vi "OP1_RISCALDO.vi"(0 "Esito 2 in":cluster{"Si":bool, "No":bool}, 1 "Esito 3 in":cluster{"Si":bool, "No":bool}, 2 "Esito 4 in":cluster{"Si":bool, "No":bool}, 3 "Esito 5 in":cluster{"Si":bool, "No":bool}, 4 "Esito 6 in":cluster{"Si":bool, "No":bool}, 5 "Esito 7 in":cluster{"Si":bool, "No":bool}, 6 "Esito 8 in":cluster{"Si":bool, "No":bool}, 7 "Esito 9 in":cluster{"Si":bool, "No":bool}, 8 "Esito 1 in":cluster{"Si":bool, "No":bool}, 9 "Tasto premuto":T1(array[ring]), 10 "Tipo specifica":string, 12 "Stato in":u16, 14 "Stato out":u16) -> (16 "Dato":string[](array[string]), 17 "ANNULLA PROVA":bool, 18 "Esito 1 out":T2, 19 "i out":i32=1, 20 "Esito 2 out":T2, 21 "Esito 3 out":T2, 22 "Esito 4 out":T2, 23 "Esito 5 out":T2, 24 "Esito 6 out":T2, 25 "Esito 7 out":T2, 26 "Esito 8 out":T2, 27 "Esito 9 out":T2)   [LabVIEW 2022 SP3]
uses:
  Labview/Globali.vi
panel:
  out "Memoria fase succ":bool
  in  "i max":i32
  in  "i":i32=1
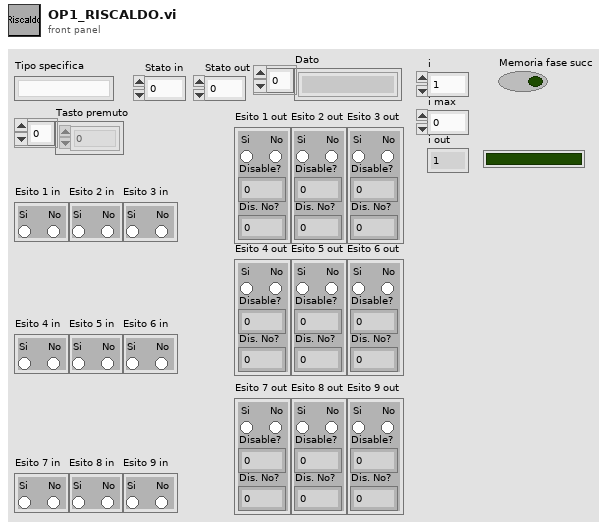
[diagram p1: front panel]
types:
  T1 = enum16{"0", "1", "2", "3", "4", "5", "6", "7", "8", "9", "A", "B", "C", "D", "E", "F", "G", "H", "I", "J", "K", "L", "M", "N", "O", "P", "Q", "R", "S", "T", "U", "V", "W", "X", "Y", "Z", "F1", "F2", "F3", "F4", "F5", "F6", "F7", "F8", "F9", "F10", "F11", "F12", "F13", "F14", "F15", "ADD", "BACK", "BACKSLASH", "CAPITAL", "COMMA", "DECIMAL", "DELETE", "DIVIDE", "DOWN", "END", "EQUALS", "ESCAPE", "GRAVE (`)", "HOME", "INSERT", "LBRACKET", "LCONTROL", "LEFT", "L ALT", "LSHIFT", "LWIN", "MINUS", "MULTIPLY", "NEXT", "NUMLOCK", "NUMPAD_0", "NUMPAD_1", "NUMPAD_2", "NUMPAD_3", "NUMPAD_4", "NUMPAD_5", "NUMPAD_6", "NUMPAD_7", "NUMPAD_8", "NUMPAD_9", "PAUSE", "PERIOD", "PRIOR (PG UP)", "RBRACKET", "RCONTROL", "RETURN", "RIGHT", "R ALT", "RSHIFT", "RWIN", "SCROLL", "SEMICOLON", "SLASH", "SPACE", "SUBTRACT", "TAB", "UP", "ENTER (num pad)", "' (quote)"}[]
  T2 = cluster{"Disable?":i16, "Si":bool, "No":bool, "Dis. No?":i16}
  T3 = cluster{"Esito 1 out":cluster{"Disable?":i16, "Si":bool, "No":bool, "Dis. No?":i16}, "Esito 2 out":cluster{"Disable?":i16, "Si":bool, "No":bool, "Dis. No?":i16}, "Esito 3 out":cluster{"Disable?":i16, "Si":bool, "No":bool, "Dis. No?":i16}, "Esito 4 out":cluster{"Disable?":i16, "Si":bool, "No":bool, "Dis. No?":i16}, "Esito 5 out":cluster{"Disable?":i16, "Si":bool, "No":bool, "Dis. No?":i16}, "Esito 6 out":cluster{"Disable?":i16, "Si":bool, "No":bool, "Dis. No?":i16}, "Esito 7 out":cluster{"Disable?":i16, "Si":bool, "No":bool, "Dis. No?":i16}, "Esito 8 out":cluster{"Disable?":i16, "Si":bool, "No":bool, "Dis. No?":i16}, "Esito 9 out":cluster{"Disable?":i16, "Si":bool, "No":bool, "Dis. No?":i16}}
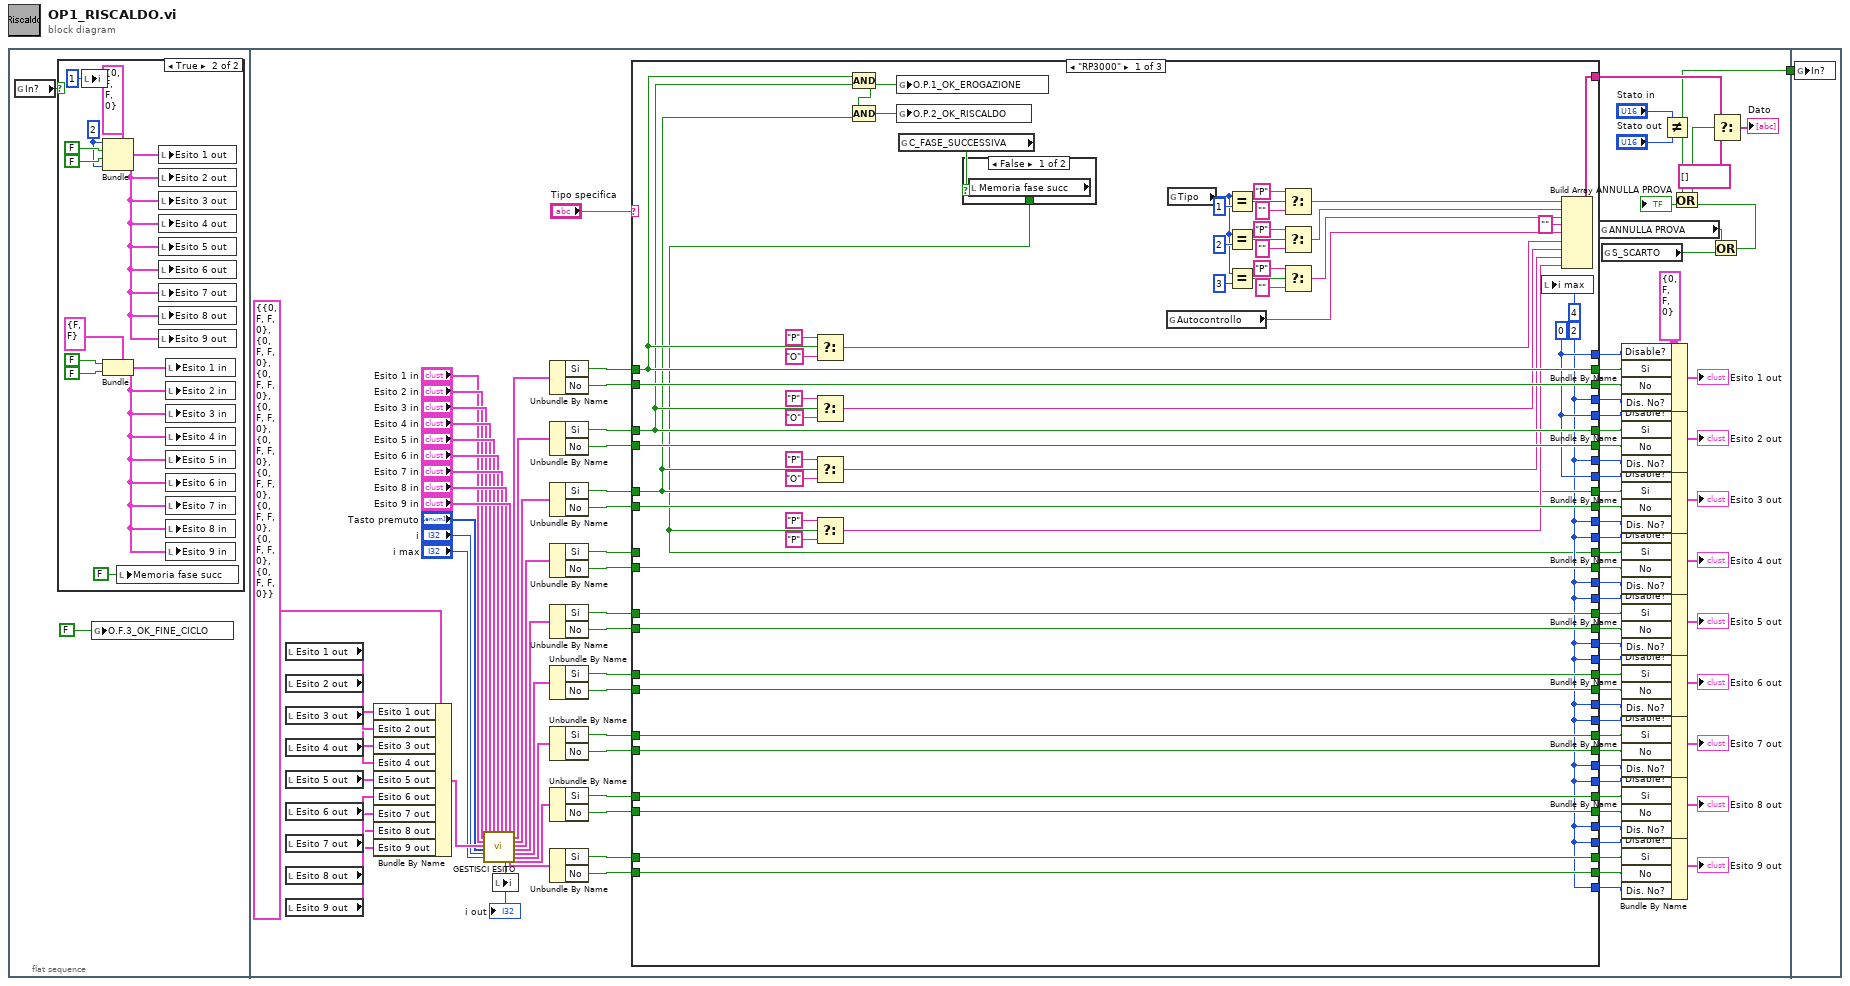
[diagram p0: block diagram]
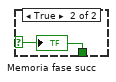
[diagram p3: hidden frame]
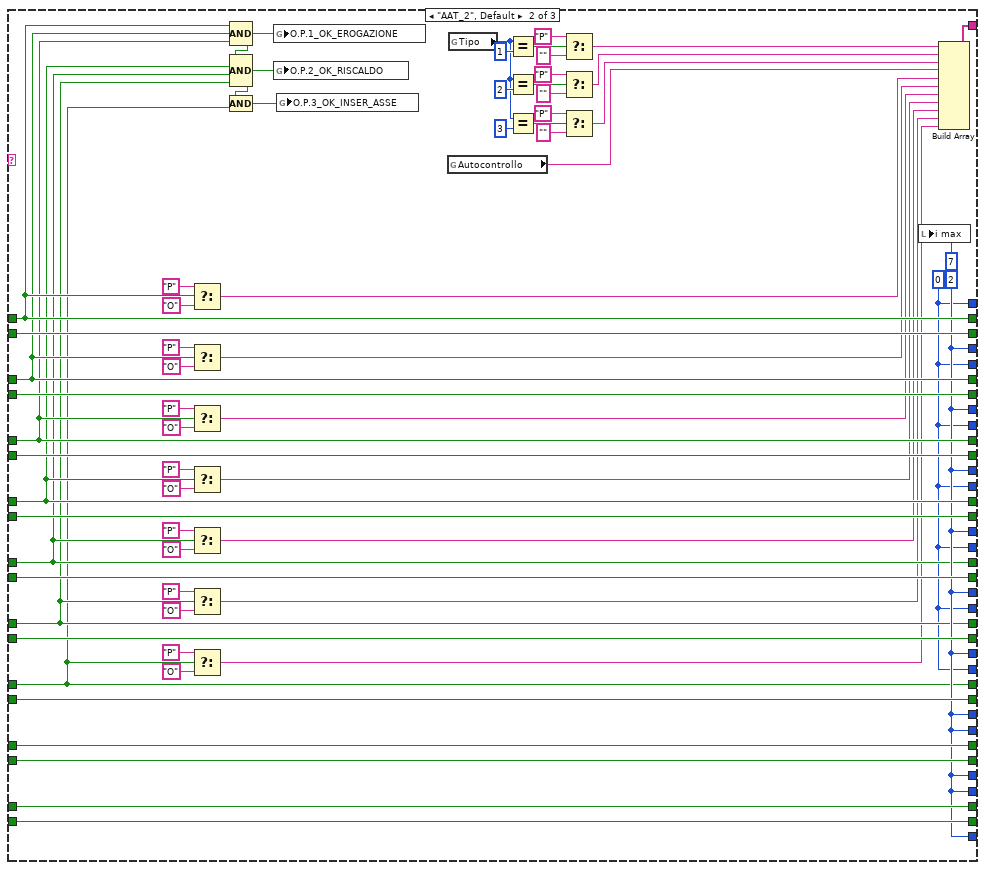
[diagram p4: hidden frame]
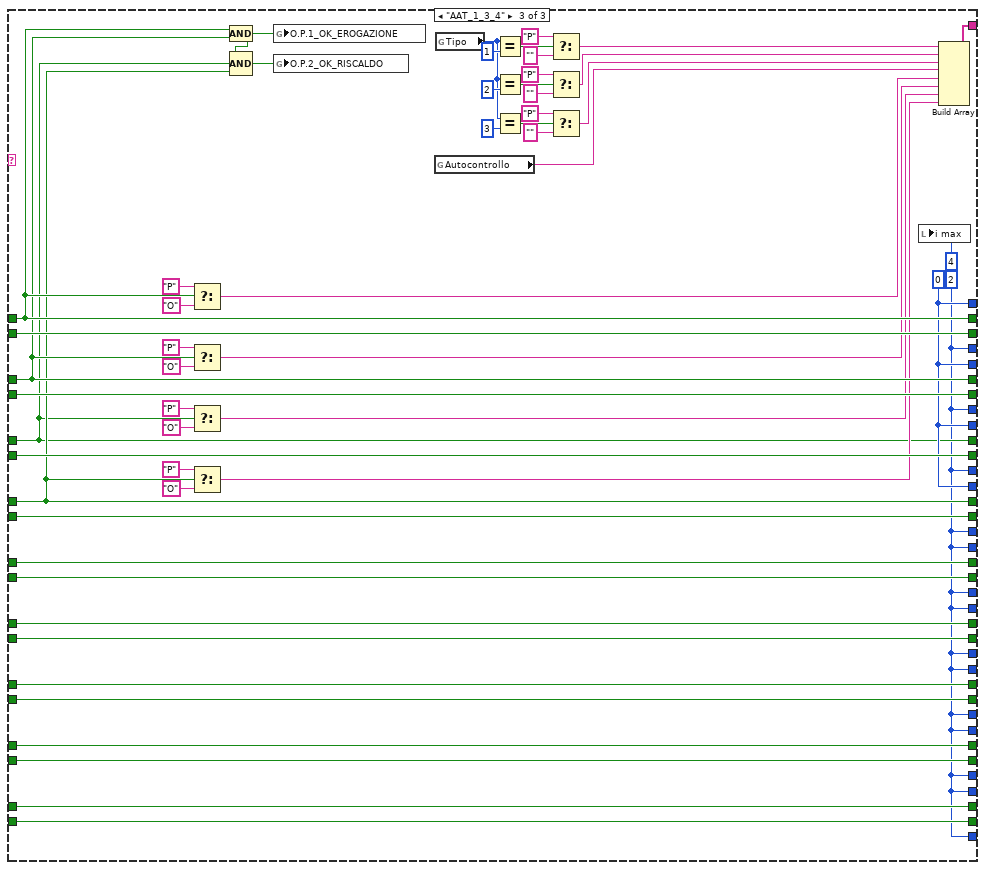
[diagram p5: hidden frame]
diagram:
  n1 = flat-sequence {
    tunnel: [w19] -> w1
    tunnel: w1 -> [w296]
    frame #0 {
      n2 = global read "Globali.vi" "In?"() -> (w3:bool)
      n3 = case shown="True" w3 {
        frame False {
        }
        frame True {
          w11 = i16 2 ("Disable?")
          n4 = local write "i"(1 ("i")) -> ()
          n5 = Bundle(cluster=T2 {"Disable?"=0, "Si"=FALSE, "No"=FALSE, "Dis. No?"=0} ("Esito 1 out"), "Disable?"=w11, "Si"=FALSE, "No"=FALSE, "Dis. No?"=w11) -> (w10:T2)
          n6 = Bundle(cluster=cluster{"Si":bool, "No":bool} {"Si"=FALSE, "No"=FALSE} ("Esito 1 in"), "Si"=FALSE, "No"=FALSE) -> (w8:cluster{"Si":bool, "No":bool})
          n7 = local write "Memoria fase succ"(FALSE ("Memoria fase succ")) -> ()
          n8 = local write "Esito 1 out"(w10) -> ()
          n9 = local write "Esito 2 out"(w10) -> ()
          n10 = local write "Esito 3 out"(w10) -> ()
          n11 = local write "Esito 4 out"(w10) -> ()
          n12 = local write "Esito 5 out"(w10) -> ()
          n13 = local write "Esito 6 out"(w10) -> ()
          n14 = local write "Esito 7 out"(w10) -> ()
          n15 = local write "Esito 8 out"(w10) -> ()
          n16 = local write "Esito 9 out"(w10) -> ()
          n17 = local write "Esito 1 in"(w8) -> ()
          n18 = local write "Esito 2 in"(w8) -> ()
          n19 = local write "Esito 3 in"(w8) -> ()
          n20 = local write "Esito 4 in"(w8) -> ()
          n21 = local write "Esito 5 in"(w8) -> ()
          n22 = local write "Esito 6 in"(w8) -> ()
          n23 = local write "Esito 7 in"(w8) -> ()
          n24 = local write "Esito 8 in"(w8) -> ()
          n25 = local write "Esito 9 in"(w8) -> ()
        }
      }
      n26 = global write "Globali.vi" "O.F.3_OK_FINE_CICLO"(FALSE ("O.F.3_OK_FINE_CICLO")) -> ()
    }
    frame #1 {
      w62 = T2 {"Disable?"=0, "Si"=FALSE, "No"=FALSE, "Dis. No?"=0} ("Esito 1 out")
      n27 = local read "Esito 1 out"() -> (w51:T2)
      n28 = local read "Esito 2 out"() -> (w50:T2)
      n29 = local read "Esito 3 out"() -> (w49:T2)
      n30 = local read "Esito 4 out"() -> (w48:T2)
      n31 = local read "Esito 5 out"() -> (w47:T2)
      n32 = local read "Esito 6 out"() -> (w46:T2)
      n33 = local read "Esito 7 out"() -> (w45:T2)
      n34 = local read "Esito 8 out"() -> (w44:T2)
      n35 = local read "Esito 9 out"() -> (w43:T2)
      n36 = Bundle By Name(cluster=T3 {"Esito 1 out"={"Disable?"=0, "Si"=FALSE, "No"=FALSE, "Dis. No?"=0}, "Esito 2 out"={"Disable?"=0, "Si"=FALSE, "No"=FALSE, "Dis. No?"=0}, "Esito 3 out"={"Disable?"=0, "Si"=FALSE, "No"=FALSE, "Dis. No?"=0}, "Esito 4 out"={"Disable?"=0, "Si"=FALSE, "No"=FALSE, "Dis. No?"=0}, "Esito 5 out"={"Disable?"=0, "Si"=FALSE, "No"=FALSE, "Dis. No?"=0}, "Esito 6 out"={"Disable?"=0, "Si"=FALSE, "No"=FALSE, "Dis. No?"=0}, "Esito 7 out"={"Disable?"=0, "Si"=FALSE, "No"=FALSE, "Dis. No?"=0}, "Esito 8 out"={"Disable?"=0, "Si"=FALSE, "No"=FALSE, "Dis. No?"=0}, "Esito 9 out"={"Disable?"=0, "Si"=FALSE, "No"=FALSE, "Dis. No?"=0}} ("Cluster"), "Esito 1 out"=w51, "Esito 2 out"=w50, "Esito 3 out"=w49, "Esito 4 out"=w48, "Esito 5 out"=w47, "Esito 6 out"=w46, "Esito 7 out"=w45, "Esito 8 out"=w44, "Esito 9 out"=w43) -> (w42:T3)
      n37 = call "GESTISCI ESITO.vi"("Esito 3 in"="Esito 3 in", "Esito 2 in"="Esito 2 in", "Esito 1 in"="Esito 1 in", "Cluster"=w42, "Tasto premuto"="Tasto premuto", "i in"="i", "i max"="i max", "Esito 4 in"="Esito 4 in", "Esito 5 in"="Esito 5 in", "Esito 6 in"="Esito 6 in", "Esito 7 in"="Esito 7 in", "Esito 8 in"="Esito 8 in", "Esito 9 in"="Esito 9 in") -> ("i out"=w20:i32, "Esito 9 in 2"=w21:cluster{"Si":bool, "No":bool}, "Esito 1 in 2"=w29:cluster{"Si":bool, "No":bool}, "Esito 2 in 2"=w28:cluster{"Si":bool, "No":bool}, "Esito 3 in 2"=w27:cluster{"Si":bool, "No":bool}, "Esito 4 in 2"=w26:cluster{"Si":bool, "No":bool}, "Esito 5 in 2"=w25:cluster{"Si":bool, "No":bool}, "Esito 6 in 2"=w24:cluster{"Si":bool, "No":bool}, "Esito 7 in 2"=w23:cluster{"Si":bool, "No":bool}, "Esito 8 in 2"=w22:cluster{"Si":bool, "No":bool})  [unwired: 5 in]
      "i out" <- w20
      n38 = local write "i"(w20) -> ()
      n39 = Unbundle By Name(w29) -> ("Si"=w86:bool, "No"=w85:bool)
      n40 = Unbundle By Name(w28) -> ("Si"=w69:bool, "No"=w70:bool)
      n41 = Unbundle By Name(w27) -> ("Si"=w71:bool, "No"=w72:bool)
      n42 = Unbundle By Name(w26) -> ("Si"=w73:bool, "No"=w74:bool)
      n43 = Unbundle By Name(w25) -> ("Si"=w75:bool, "No"=w76:bool)
      n44 = Unbundle By Name(w24) -> ("Si"=w77:bool, "No"=w78:bool)
      n45 = Unbundle By Name(w23) -> ("Si"=w79:bool, "No"=w80:bool)
      n46 = Unbundle By Name(w22) -> ("Si"=w81:bool, "No"=w82:bool)
      n47 = Unbundle By Name(w21) -> ("Si"=w83:bool, "No"=w84:bool)
      n48 = case shown="\"RP3000\"" "Tipo specifica" {
        tunnel: [w152 w214 w272] -> w66
        tunnel: [w146 w198 w264] -> w113
        tunnel: [w146 w198 w264] -> w112
        tunnel: [w146 w198 w264] -> w111
        tunnel: [w143 w198 w264] -> w110
        tunnel: [w143 w198 w261] -> w109
        tunnel: [w143 w198 w261] -> w108
        tunnel: [w143 w198 w261] -> w107
        tunnel: [w143 w215 w261] -> w106
        tunnel: [w143 w215 w261] -> w105
        tunnel: [w161 w228 w281] -> w104
        tunnel: [w160 w227 w280] -> w103
        tunnel: [w159 w226 w279] -> w102
        tunnel: [w162 w229 w282] -> w101
        tunnel: [w145 w219 w262] -> w100
        tunnel: [w177 w242 w295] -> w99
        tunnel: [w141 w217 w263] -> w98
        tunnel: [w176 w241 w294] -> w97
        tunnel: [w144 w208 w267] -> w96
        tunnel: [w175 w240 w293] -> w95
        tunnel: [w174 w202 w266] -> w94
        tunnel: [w173 w239 w292] -> w93
        tunnel: [w172 w201 w265] -> w92
        tunnel: [w171 w238 w291] -> w91
        tunnel: [w170 w237 w290] -> w90
        tunnel: [w169 w236 w289] -> w89
        tunnel: [w168 w235 w288] -> w88
        tunnel: [w167 w234 w287] -> w87
        tunnel: w86 -> [w161 w228 w281]
        tunnel: w85 -> [w160 w227 w280]
        tunnel: w84 -> [w167 w234 w287]
        tunnel: w83 -> [w168 w235 w288]
        tunnel: w82 -> [w169 w236 w289]
        tunnel: w81 -> [w170 w237 w290]
        tunnel: w80 -> [w171 w238 w291]
        tunnel: w79 -> [w172 w201 w265]
        tunnel: w78 -> [w173 w239 w292]
        tunnel: w77 -> [w174 w202 w266]
        tunnel: w76 -> [w175 w240 w293]
        tunnel: w75 -> [w144 w208 w267]
        tunnel: w74 -> [w176 w241 w294]
        tunnel: w73 -> [_ w217 w263]
        tunnel: w72 -> [w177 w242 w295]
        tunnel: w71 -> [w145 w219 w262]
        tunnel: w70 -> [w162 w229 w282]
        tunnel: w69 -> [w159 w226 w279]
        tunnel: [w143 w215 w261] -> w61
        tunnel: [w143 w215 w261] -> w60
        tunnel: [w143 w215 w261] -> w59
        tunnel: [w143 w215 w261] -> w58
        tunnel: [w143 w215 w261] -> w57
        tunnel: [w143 w215 w261] -> w56
        tunnel: [w143 w215 w261] -> w55
        tunnel: [w143 w215 w261] -> w54
        tunnel: [w143 w215 w261] -> w53
        frame "RP3000" {
          w143 = 2
          w146 = 0
          n49 = Select(t="P", s=w161, f="O") -> (s? t:f=w148:string)
          n50 = Select(t="P", s=w159, f="O") -> (s? t:f=w149:string)
          n51 = Select(t="P", s=w145, f="O") -> (s? t:f=w150:string)
          n52 = Compound Arithmetic op=AND(w161, w159) -> (w154:bool)
          n53 = Compound Arithmetic op=AND(w154, w145) -> (w153:bool)
          n54 = global write "Globali.vi" "O.P.1_OK_EROGAZIONE"(w154) -> ()
          n55 = global write "Globali.vi" "O.P.2_OK_RISCALDO"(w153) -> ()
          n56 = global read "Globali.vi" "C_FASE_SUCCESSIVA"() -> (w142:bool)
          n57 = case shown="False" w142 {
            selector: w142 -> [_ w179]
            tunnel: [w178 w179] -> w141
            frame False {
              n58 = local read "Memoria fase succ"() -> (w178:bool)
            }
            frame True {
              "Memoria fase succ" <- w179
            }
          }
          n59 = Select(t="P", s=w141, f="P") -> (s? t:f=w151:string)
          n60 = global read "Globali.vi" "Autocontrollo"() -> (w127:string)
          n61 = global read "Globali.vi" "Tipo"() -> (w128:i16)
          n62 = Equal?(x=w128, y=i16 1) -> (x = y?=w137:bool)
          n63 = Equal?(x=w128, y=i16 2) -> (x = y?=w133:bool)
          n64 = Equal?(x=w128, y=i16 3) -> (x = y?=w132:bool)
          n65 = Select(t="P", s=w137, f="") -> (s? t:f=w124:string)
          n66 = Select(t="P", s=w133, f="") -> (s? t:f=w125:string)
          n67 = Select(t="P", s=w132, f="") -> (s? t:f=w126:string)
          n68 = local write "i max"(4) -> ()
          n69 = Build Array(w124, w125, w126, "" ("element"), w127, w148, w149, w150, w151) -> (w152:string[])
        }
        frame "AAT_2", Default {
          w215 = 2
          w198 = 0
          n70 = Select(t="P", s=w228, f="O") -> (s? t:f=w209:string)
          n71 = Select(t="P", s=w226, f="O") -> (s? t:f=w210:string)
          n72 = Select(t="P", s=w219, f="O") -> (s? t:f=w211:string)
          n73 = Select(t="P", s=w217, f="O") -> (s? t:f=w212:string)
          n74 = Select(t="P", s=w208, f="O") -> (s? t:f=w213:string)
          n75 = Select(t="P", s=w202, f="O") -> (s? t:f=w200:string)
          n76 = Select(t="P", s=w201, f="O") -> (s? t:f=w199:string)
          n77 = Compound Arithmetic op=AND(w228, w226, w219) -> (w218:bool)
          n78 = Compound Arithmetic op=AND(w218, w217, w208, w202) -> (w216:bool)
          n79 = Compound Arithmetic op=AND(w216, w201) -> (w207:bool)
          n80 = global write "Globali.vi" "O.P.1_OK_EROGAZIONE"(w218) -> ()
          n81 = global write "Globali.vi" "O.P.2_OK_RISCALDO"(w216) -> ()
          n82 = global write "Globali.vi" "O.P.3_OK_INSER_ASSE"(w207) -> ()
          n83 = global read "Globali.vi" "Autocontrollo"() -> (w180:string)
          n84 = global read "Globali.vi" "Tipo"() -> (w184:i16)
          n85 = Equal?(x=w184, y=i16 1) -> (x = y?=w193:bool)
          n86 = Equal?(x=w184, y=i16 2) -> (x = y?=w189:bool)
          n87 = Equal?(x=w184, y=i16 3) -> (x = y?=w188:bool)
          n88 = Select(t="P", s=w193, f="") -> (s? t:f=w183:string)
          n89 = Select(t="P", s=w189, f="") -> (s? t:f=w182:string)
          n90 = Select(t="P", s=w188, f="") -> (s? t:f=w181:string)
          n91 = local write "i max"(7) -> ()
          n92 = Build Array(w183, w182, w181, w180, w209, w210, w211, w212, w213, w200, w199) -> (w214:string[])
        }
        frame "AAT_1_3_4" {
          w261 = 2
          w264 = 0
          n93 = Select(t="P", s=w281, f="O") -> (s? t:f=w268:string)
          n94 = Select(t="P", s=w279, f="O") -> (s? t:f=w269:string)
          n95 = Select(t="P", s=w262, f="O") -> (s? t:f=w270:string)
          n96 = Select(t="P", s=w263, f="O") -> (s? t:f=w271:string)
          n97 = Compound Arithmetic op=AND(w281, w279) -> (w274:bool)
          n98 = Compound Arithmetic op=AND(w274, w262, w263) -> (w273:bool)
          n99 = global write "Globali.vi" "O.P.1_OK_EROGAZIONE"(w274) -> ()
          n100 = global write "Globali.vi" "O.P.2_OK_RISCALDO"(w273) -> ()
          n101 = global read "Globali.vi" "Autocontrollo"() -> (w243:string)
          n102 = global read "Globali.vi" "Tipo"() -> (w247:i16)
          n103 = Equal?(x=w247, y=i16 1) -> (x = y?=w256:bool)
          n104 = Equal?(x=w247, y=i16 2) -> (x = y?=w252:bool)
          n105 = Equal?(x=w247, y=i16 3) -> (x = y?=w251:bool)
          n106 = Select(t="P", s=w256, f="") -> (s? t:f=w246:string)
          n107 = Select(t="P", s=w252, f="") -> (s? t:f=w245:string)
          n108 = Select(t="P", s=w251, f="") -> (s? t:f=w244:string)
          n109 = local write "i max"(4) -> ()
          n110 = Build Array(w246, w245, w244, w243, w268, w269, w270, w271) -> (w272:string[])
        }
      }
      n111 = global read "Globali.vi" "ANNULLA PROVA"() -> (w16:bool)
      n112 = global read "Globali.vi" "S_SCARTO"() -> (w17:bool)
      n113 = Bundle By Name(cluster=w62, "Disable?"=w113, "Si"=w104, "No"=w103, "Dis. No?"=w61) -> (→"Esito 1 out":T2)
      n114 = Bundle By Name(cluster=w62, "Disable?"=w112, "Si"=w102, "No"=w101, "Dis. No?"=w60) -> (→"Esito 2 out":T2)
      n115 = Bundle By Name(cluster=w62, "Disable?"=w111, "Si"=w100, "No"=w99, "Dis. No?"=w59) -> (→"Esito 3 out":T2)
      n116 = Bundle By Name(cluster=w62, "Disable?"=w110, "Si"=w98, "No"=w97, "Dis. No?"=w58) -> (→"Esito 4 out":T2)
      n117 = Bundle By Name(cluster=w62, "Disable?"=w109, "Si"=w96, "No"=w95, "Dis. No?"=w57) -> (→"Esito 5 out":T2)
      n118 = Bundle By Name(cluster=w62, "Disable?"=w108, "Si"=w94, "No"=w93, "Dis. No?"=w56) -> (→"Esito 6 out":T2)
      n119 = Bundle By Name(cluster=w62, "Disable?"=w107, "Si"=w92, "No"=w91, "Dis. No?"=w55) -> (→"Esito 7 out":T2)
      n120 = Bundle By Name(cluster=w62, "Disable?"=w106, "Si"=w90, "No"=w89, "Dis. No?"=w54) -> (→"Esito 8 out":T2)
      n121 = Bundle By Name(cluster=w62, "Disable?"=w105, "Si"=w88, "No"=w87, "Dis. No?"=w53) -> (→"Esito 9 out":T2)
      n122 = Not Equal?(x="Stato in", y="Stato out") -> (x != y?=w19:bool)
      n123 = Or(x=w16, y=w17) -> (x .or. y?=w15:bool)
      "ANNULLA PROVA" <- w15
      n124 = Or(x=w19, y=w15) -> (x .or. y?=w18:bool)
      n125 = Select(t=w66, s=w18, f=string[] [] ("Dato")) -> (s? t:f=→"Dato":string[])
    }
    frame #2 {
      n126 = global write "Globali.vi" "In?"(w296) -> ()
    }
  }
